vi "__init__.vi"(6 "init_value":T1, 7 "Lock-In Amplifier":refnum<class "Lock-In Amplifier.lvclass">, 8 "error in":errorcluster, 9 "Function Generator":refnum<class "Function Generator.lvclass">, 10 "Picomotor":refnum<class "Picomotor.lvclass">, 11 "PZT":refnum<class "PZT.lvclass">) -> (0 "error out":errorcluster, 3 "Coarse Approach.lvclass":refnum<class "Coarse Approach.lvclass">)   [LabVIEW 2020, in "Coarse Approach.lvclass"]
uses:
  Coarse Approach.lvclass
  Lock-In Amplifier/Lock-In Amplifier.lvclass
  PZT/PZT.lvclass
  Function Generator/Function Generator.lvclass
  Picomotor/Picomotor.lvclass
  Coarse Approach.lvclass/Coarse Approach.ctl
  <vilib>/Analysis/baseanly.llb/Mean (DBL).vi
  <vilib>/Analysis/NI_AALBase.lvlib
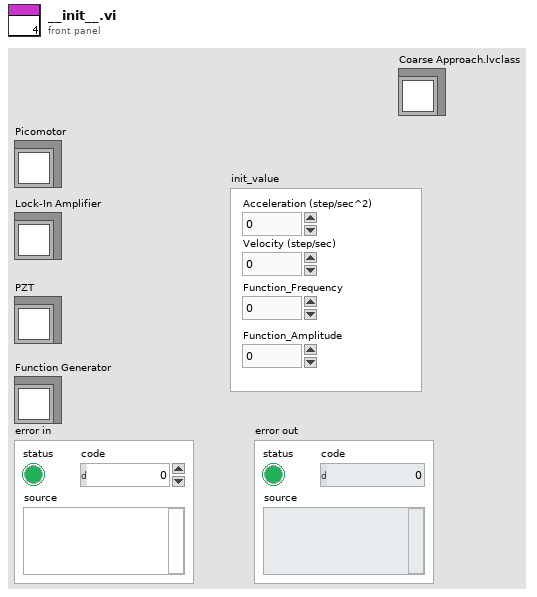
[diagram p1: front panel]
types:
  T1 = cluster{"Function_Amplitude":dbl, "Acceleration (step/sec^2)":i32, "Velocity (step/sec)":i32, "Function_Frequency":dbl}
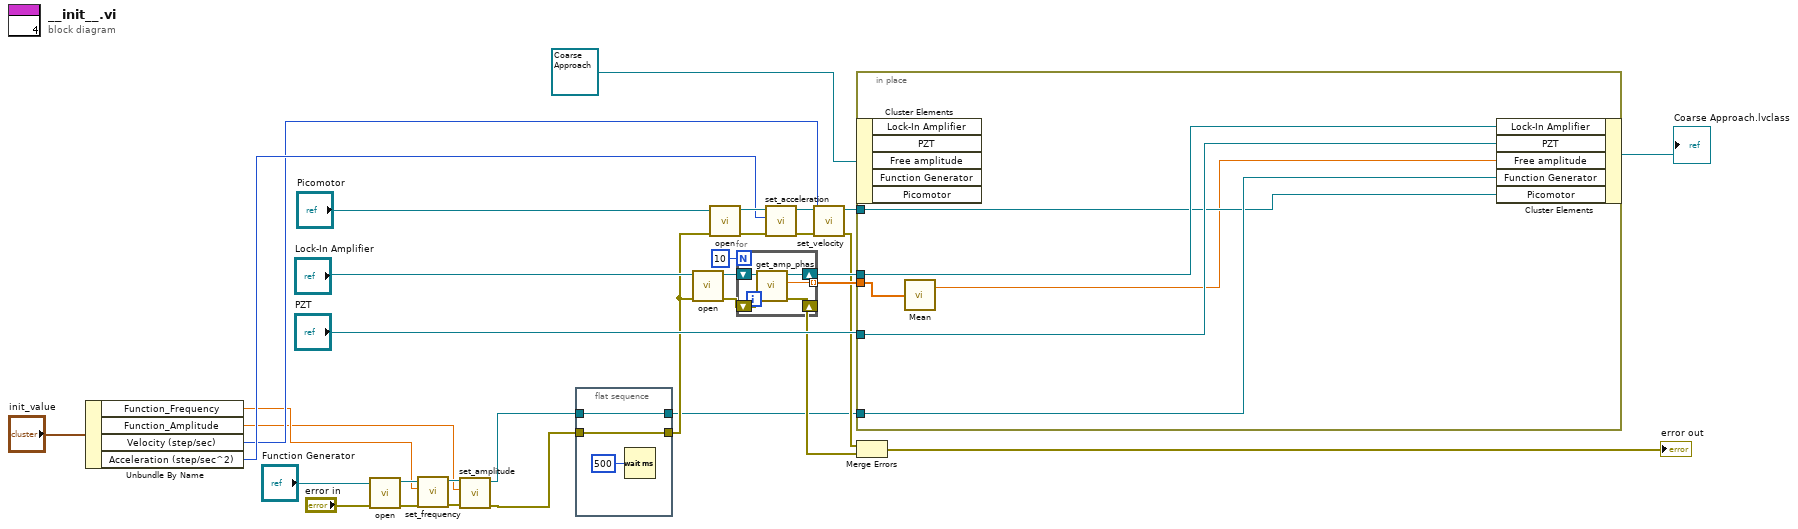
[diagram p0: block diagram]
diagram:
  n1 = Unbundle By Name("init_value") -> ("Function_Frequency"=w7:dbl, "Function_Amplitude"=w6:dbl, "Velocity (step/sec)"=w8:i32, "Acceleration (step/sec^2)"=w9:i32)
  n2 = call-dynamic "open.vi"("error in (no error)"="error in", "Function Generator in"="Function Generator") -> ("error out"=w12:errorcluster, "Function Generator out"=w14:refnum<class "Function Generator.lvclass">)  [unwired: 8 in]
  n3 = call-dynamic "set_frequency.vi"("error in (no error)"=w12, "Frequency"=w7, "Function Generator in"=w14) -> ("error out"=w11:errorcluster, "Function Generator out"=w13:refnum<class "Function Generator.lvclass">)  [unwired: 7 in]
  n4 = call-dynamic "set_amplitude.vi"("error in (no error)"=w11, "Amplitude"=w6, "Function Generator in"=w13) -> ("error out"=w5:errorcluster, "Function Generator out"=w4:refnum<class "Function Generator.lvclass">)  [unwired: 7 in]
  n5 = flat-sequence {
    tunnel: w5 -> [w36]
    tunnel: [w36] -> w16
    tunnel: w4 -> [w34]
    tunnel: [w34] -> w3
    frame #0 {
      n6 = Wait (ms)(milliseconds to wait=u32 500) -> ()  [unwired: 1 out]
    }
  }
  n7 = call-dynamic "open.vi"("error in (no error)"=w16, "Instrument in"="Lock-In Amplifier") -> ("error out"=w31:errorcluster, "Instrument out"=w32:refnum<class "Lock-In Amplifier.lvclass">)  [unwired: 8 in]
  n8 = call-dynamic "open.vi"("error in (no error)"=w16, "Instrument in"="Picomotor") -> ("error out"=w19:errorcluster, "Instrument out"=w22:refnum<class "Picomotor.lvclass">)  [unwired: 8 in]
  n9 = for {
    N: 10 -> [_]
    tunnel: [w38] -> w27 mode=indexing
    shift-right: [w39] -> w28
    shift-left: w32 -> [w41]
    shift-right: [w37] -> w17
    shift-left: w31 -> [w40]
    n10 = call-dynamic "get_amp_phas.vi"("error in (no error)"=w40, "Lock-In Amplifier in"=w41) -> ("error out"=w37:errorcluster, "Amplitude (V rms)"=w38:dbl, "Lock-In Amplifier out"=w39:refnum<class "Lock-In Amplifier.lvclass">)  [unwired: 6 in, 1 out]
  }
  n11 = call-dynamic "set_acceleration.vi"("error in (no error)"=w19, "Acceleration (steps/sec^2)"=w9, "Picomotor in"=w22) -> ("error out"=w18:errorcluster, "Picomotor out"=w21:refnum<class "Picomotor.lvclass">)  [unwired: 7 in]
  n12 = call-dynamic "set_velocity.vi"("error in (no error)"=w18, "Velocity (steps/sec)"=w8, "Picomotor in"=w21) -> ("error out"=w15:errorcluster, "Picomotor out"=w20:refnum<class "Picomotor.lvclass">)  [unwired: 7 in]
  n13 = in-place {
    in-place-border: w20 -> [w44]
    in-place-border: w28 -> [w47]
    in-place-border: w27 -> [w43]
    in-place-border: "PZT" -> [w46]
    in-place-border: w3 -> [w45]
    n14 = in-place-cluster #1(refnum<class "Coarse Approach.lvclass"> refnum ("Coarse Approach.lvclass")) -> ()  [unwired: 5 out]
    n15 = call-poly <vilib>:"Mean.vi"("X"=w43) -> ("mean"=w42:dbl)  [unwired: 1 out]
    n16 = in-place-cluster #1("Lock-In Amplifier"=w47, "PZT"=w46, "Free amplitude"=w42, "Function Generator"=w45, "Picomotor"=w44) -> (→"Coarse Approach.lvclass":refnum<class "Coarse Approach.lvclass">)
  }
  n17 = Merge Errors(w15, w17) -> (→"error out":errorcluster)
